vi "Test_Code.vi"() -> ()   [LabVIEW 2015]
uses:
  Serial - Settings.ctl
  Serial - XON-XOFF Characters.ctl
  Serial - ASCII Characters.ctl
  <vilib>/Instr/_visa.llb/Select Event Type.ctl
  <vilib>/Instr/_visa.llb/VISA Configure Serial Port (Instr).vi
  Global 5.vi
  <vilib>/Utility/NIReport.llb/NI_report.lvclass
  <instrlib>/Agilent N6700 Series/Agilent N6700 Series.lvlib
  <vilib>/addons/_office/NI_ReportGenerationToolkit.lvlib
panel:
  in  "report file path":path=path "C:/Users/Tulio/Documents/Testes/Backup excel/backup excel.xlsx"
  out "Hour":i32
  out "Minute":i32
  out "Second":i32
  out "Fractional Second":dbl format="%#.4g"
  in  "Negative Voltage Limit (0.0 volts)":dbl format="%^.3e"
  out "Waveform Graph":dbl[](graph)
  out "Count":i32
  out "read buffer":string
  in  "Read Count":u32=1000
  out "Action":string
  in  "Termination Character":u8=10 format="%.0x"
  in  "End Write on Termination Character?":bool=TRUE
  in  "VISA resource name 2":refnum<visa-resource-name>="COM27"
  in  "XON/XOFF Characters":T1={"XON"=enum."DC1", "XOFF"=enum."DC3"}
  in  "Serial Settings":T3={"baud rate"=9600, "data bits"=8, "parity"=enum."None", "stop bits"=10, "flow control"=0} {"flow control" items=["None"=0, "XON/XOFF"=1, "RTS/CTS"=2, "DTR/DSR"=4]; "stop bits" items=["1.0"=10, "1.5"=15, "2.0"=20]; "data bits" min=5 max=8 step=1; "baud rate" items=["75"=75, "110"=110, "134"=134, "150"=150, "300"=300, "600"=600, "1200"=1200, "1800"=1800, "2400"=2400, "4800"=4800, "7200"=7200, "9600"=9600, "14400"=14400, "19200"=19200, "28800"=28800, "38400"=38400, "56000"=56000, "57600"=57600, "115200"=115200, "128000"=128000, "230400"=230400]}
  in  "End Read on Termination Character?":bool=TRUE
  in  "Start":bool
  in  "Priority (1: Voltage)":i32(ring) items=["Voltage"=1, "Current"=0]
  out "Current Measurement":dbl format="%^.3e"
  in  "Positive Voltage Limit  (5.0 V)":dbl=5.0 format="%^.3e"
  in  "Channel Name (1)":string="4"
  in  "VISA resource name":refnum<visa-resource-name>="USB0::0x0957::0x0F07::MY53002228::INSTR"
  in  "stop":bool
  # "SERIAL"
  # "POWER ANALYZER"
  # "EXCEL"
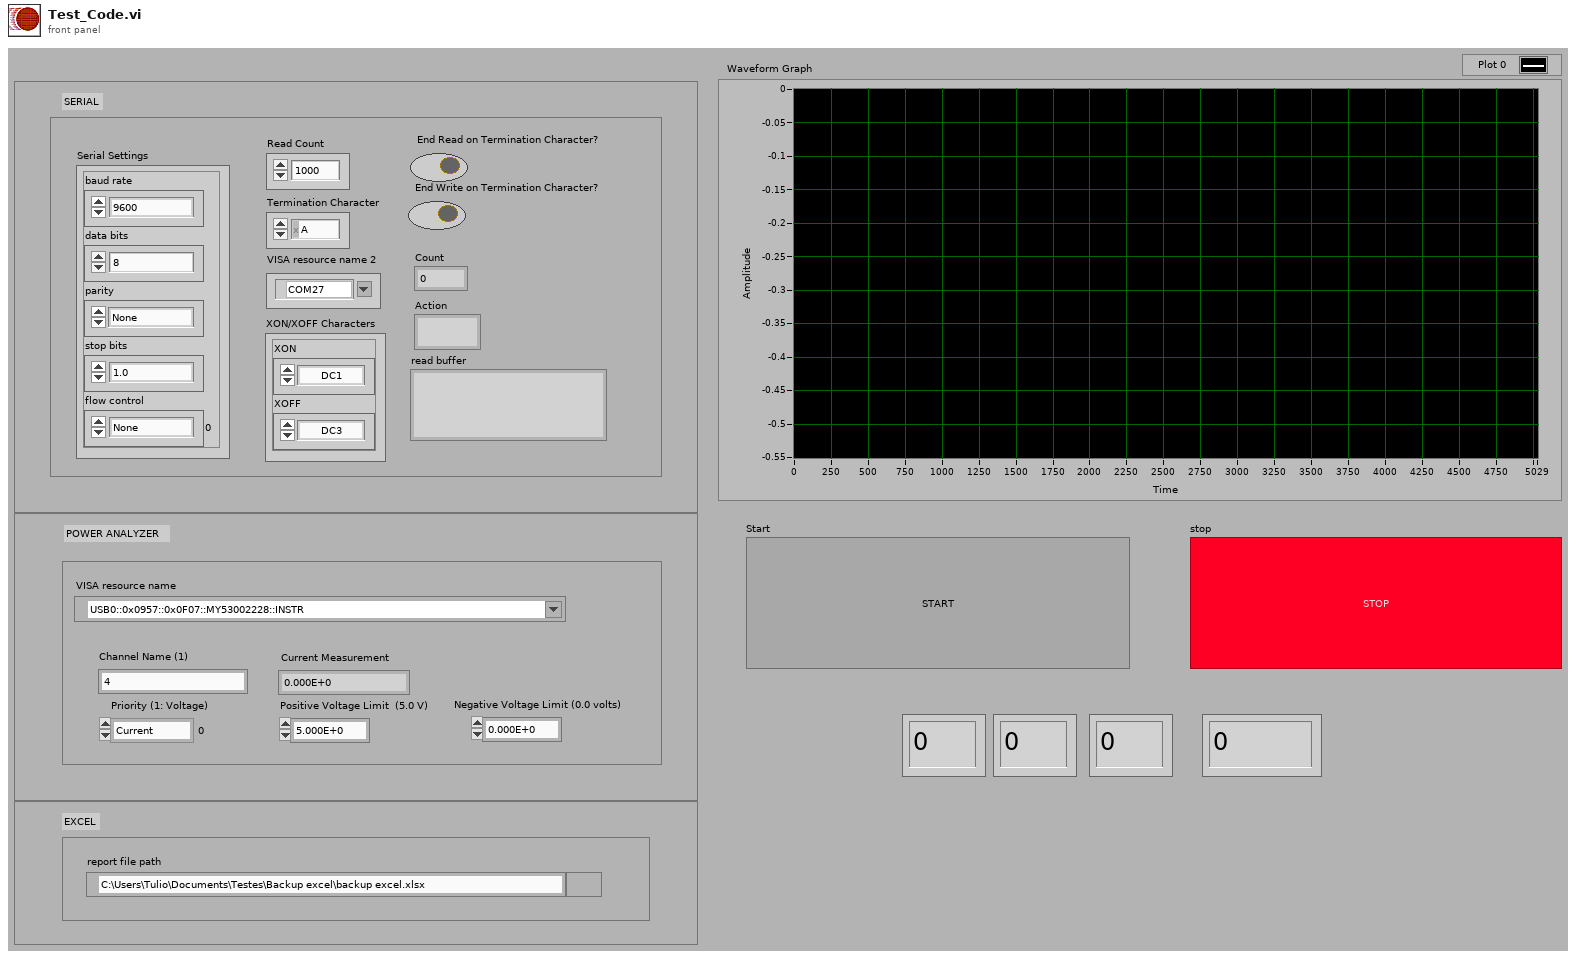
[diagram p1: front panel]
types:
  T1 = typedef "Serial - XON-XOFF Characters.ctl" = cluster{"XON":T2, "XOFF":T2}
  T2 = typedef "Serial - ASCII Characters.ctl" = enum16{"NUL", "SOH", "STX", "ETX", "EOT", "ENQ", "ACK", "BEL", "BS", "HT", "LF", "VT", "FF", "CR", "SO", "SI", "DLE", "DC1", "DC2", "DC3", "DC4", "NAK", "SYN", "ETB", "CAN", "EM", "SUB", "ESC", "FS", "GS", "RS", "US", "SP", "!", "\"", "#", "$", "%", "&", "'", "(", ")", "*", "+", ",", "- (-)", ".", "/", "0", "1", "2", "3", "4", "5", "6", "7", "8", "9", ":", ";", "<", "=", ">", "?", "@", "A", "B", "C", "D", "E", "F", "G", "H", "I", "J", "K", "L", "M", "N", "O", "P", "Q", "R", "S", "T", "U", "V", "W", "X", "Y", "Z", "[", "\\", "]", "^", "_", "`", "a", "b", "c", "d", "e", "f", "g", "h", "i", "j", "k", "l", "m", "n", "o", "p", "q", "r", "s", "t", "u", "v", "w", "x", "y", "z", "{", "|", "}", "~"}
  T3 = typedef "Serial - Settings.ctl" = cluster{"baud rate":u32, "data bits":u16, "parity":enum16{"None", "Odd", "Even", "Mark", "Space"}, "stop bits":u16, "flow control":u16}
  T4 = enum16{"Standard Report", "HTML", "Word", "Excel"}
  T5 = cluster{"Start":bool, "Pause":bool, "Reset":bool}
  T6 = typedef "Select Event Type.ctl" = u32
  T7 = typedef "LVDateTimeRec.ctl" = cluster{"fractional second":dbl, "second":i32, "minute":i32, "hour":i32, "day of month":i32, "month":i32, "year":i32, "day of week":i32, "day of year":i32, "DST":i32}
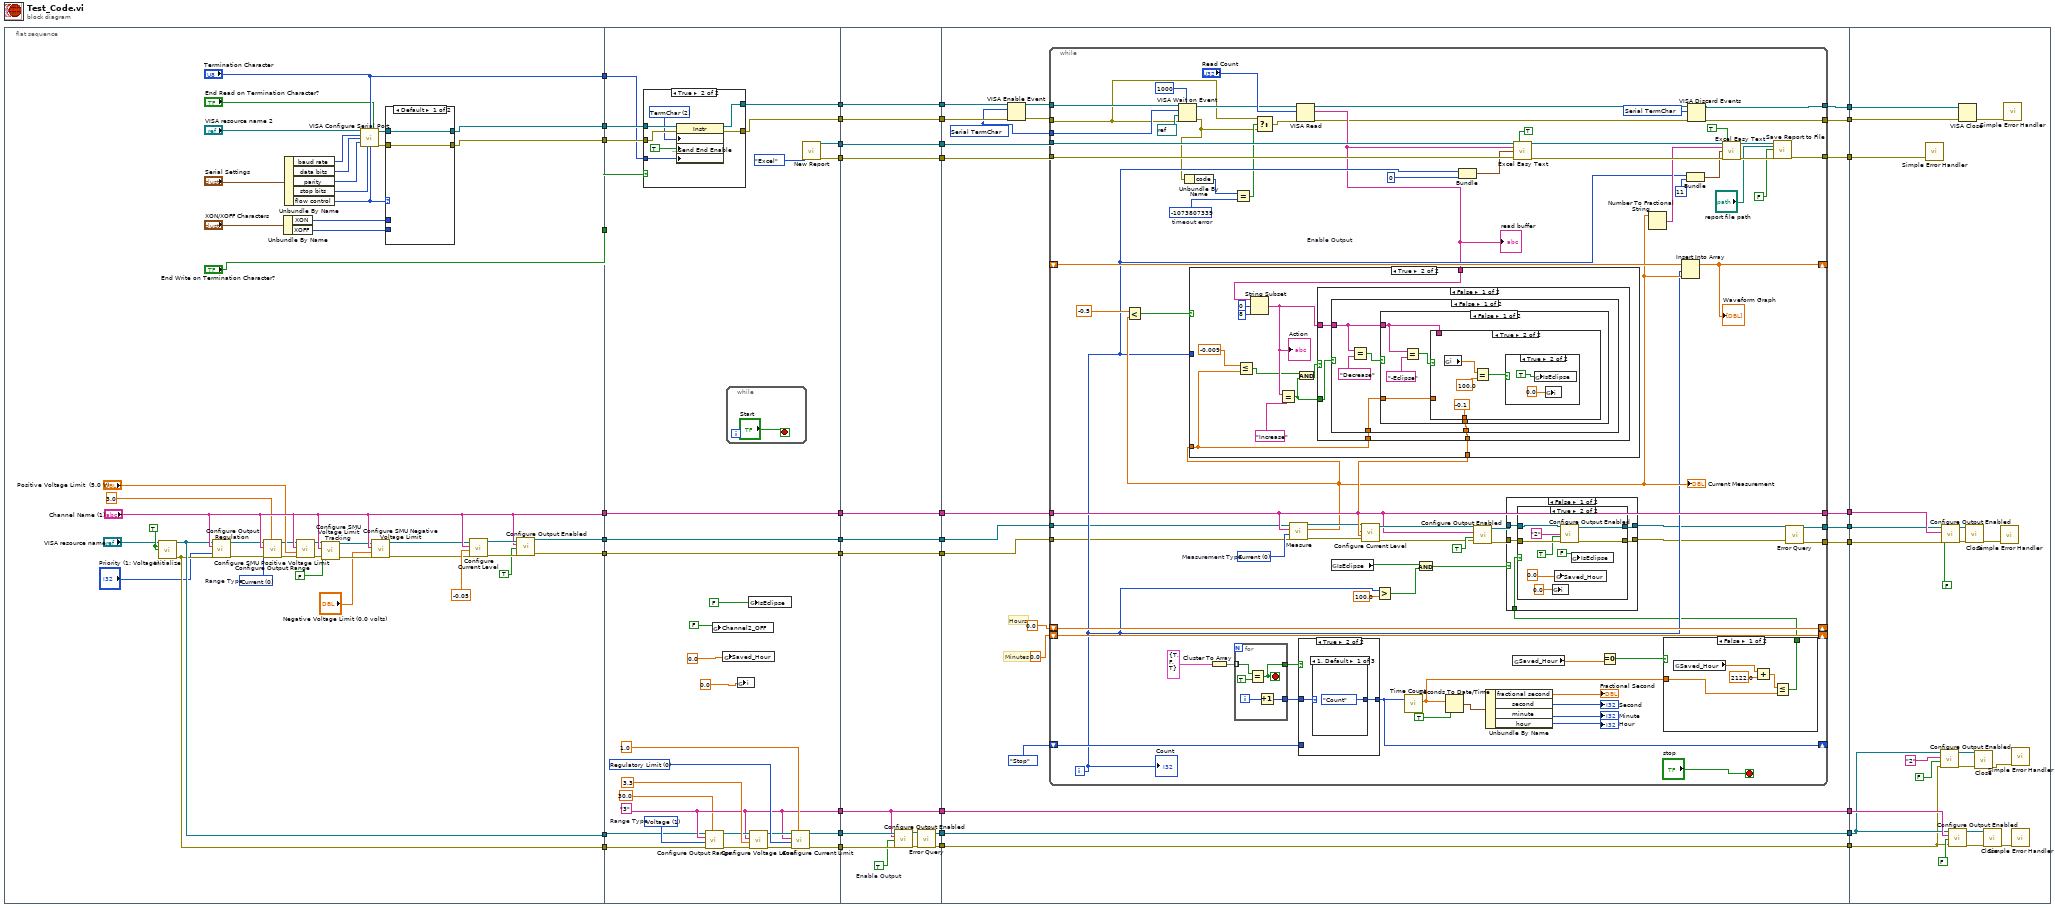
[diagram p0: block diagram]
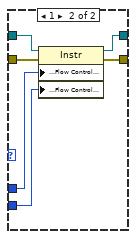
[diagram p2: hidden frame]
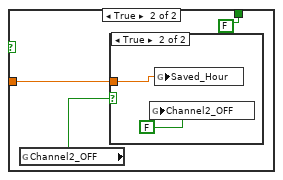
[diagram p4: hidden frame]
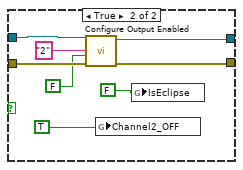
[diagram p7: hidden frame]
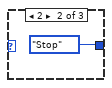
[diagram p9: hidden frame]
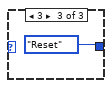
[diagram p10: hidden frame]
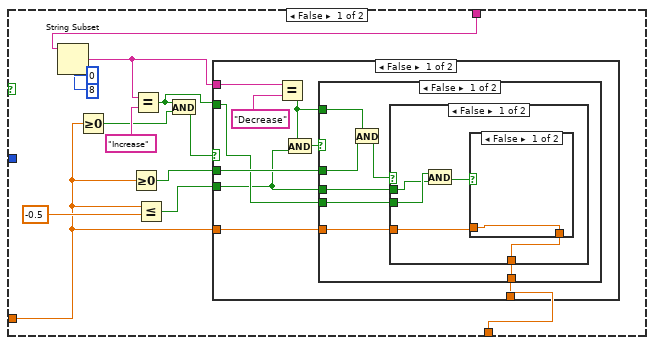
[diagram p11: hidden frame]
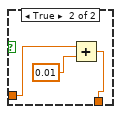
[diagram p12: hidden frame]
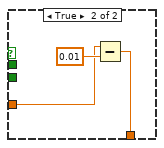
[diagram p13: hidden frame]
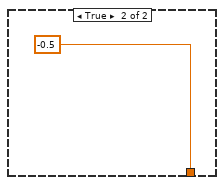
[diagram p14: hidden frame]
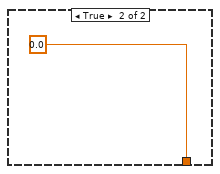
[diagram p15: hidden frame]
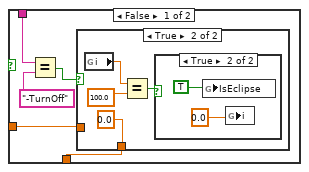
[diagram p16: hidden frame]
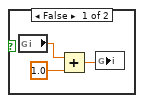
[diagram p18: hidden frame]
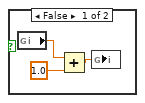
[diagram p19: hidden frame]
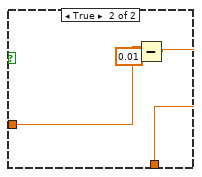
[diagram p20: hidden frame]
diagram:
  n1 = flat-sequence {
    tunnel: ["Channel Name (1)"] -> w38
    tunnel: [w80] -> w37
    tunnel: [w79] -> w36
    tunnel: [w72] -> w35
    tunnel: [w71] -> w34
    tunnel: [w76] -> w25
    tunnel: [w75] -> w24
    tunnel: ["End Write on Termination Character?"] -> w23
    tunnel: ["Termination Character"] -> w22
    tunnel: [w98] -> w20
    tunnel: [w120] -> w18
    tunnel: w38 -> [w120]
    tunnel: [w119] -> w16
    tunnel: w37 -> [w119]
    tunnel: [w118] -> w14
    tunnel: w36 -> [w118]
    tunnel: w35 -> [w99]
    tunnel: w34 -> [w101]
    tunnel: [w109] -> w11
    tunnel: w25 -> [w108]
    tunnel: w24 -> [w107]
    tunnel: w23 -> [w106]
    tunnel: w22 -> [w105]
    tunnel: [w97] -> w9
    tunnel: [w103] -> w7
    tunnel: [w102] -> w5
    tunnel: [w96] -> w2
    tunnel: [w95] -> w1
    tunnel: w20 -> [w145]
    tunnel: [w145] -> w19
    tunnel: w18 -> [w144]
    tunnel: [w144] -> w17
    tunnel: w16 -> [w143]
    tunnel: [w143] -> w15
    tunnel: w14 -> [w142]
    tunnel: [w142] -> w13
    tunnel: [w137] -> w12
    tunnel: w11 -> [w131]
    tunnel: [w131] -> w10
    tunnel: w9 -> [w141]
    tunnel: [w141] -> w8
    tunnel: w7 -> [w140]
    tunnel: [w140] -> w6
    tunnel: w5 -> [w139]
    tunnel: [w139] -> w4
    tunnel: [w138] -> w3
    tunnel: w2 -> [w134]
    tunnel: w1 -> [w133]
    tunnel: w19 -> [w151]
    tunnel: w17 -> [w167]
    tunnel: w15 -> [w166]
    tunnel: w13 -> [w165]
    tunnel: [w164] -> w33
    tunnel: [w163] -> w32
    tunnel: [w162] -> w31
    tunnel: [w161] -> w30
    tunnel: [w160] -> w29
    tunnel: w12 -> [w160]
    tunnel: w10 -> [w159]
    tunnel: [w159] -> w28
    tunnel: [w146] -> w27
    tunnel: [w158] -> w26
    tunnel: w8 -> [w150]
    tunnel: w6 -> [w154]
    tunnel: w4 -> [w153]
    tunnel: [w152] -> w21
    tunnel: w3 -> [w161]
    tunnel: w26 -> [w401]
    tunnel: w27 -> [w402]
    tunnel: w28 -> [w404]
    tunnel: w29 -> [w396]
    tunnel: w30 -> [w397]
    tunnel: w31 -> [w409]
    tunnel: w32 -> [w392]
    tunnel: w33 -> [w391]
    tunnel: w21 -> [w393]
    frame #0 {
      w63 = TRUE ("Reset? (T: Yes)")
      w62 = 0 items=["Voltage"=1, "Current"=0]  # Range Type
      n2 = call <instrlib>:"Initialize.vi"("VISA resource name"="VISA resource name", "ID Query? (T: Yes)"=w63, "Reset? (T: Yes)"=w63) -> ("VISA resource name out"=w72:refnum<visa-resource-name>, "error out"=w71:errorcluster)  [unwired: 11 in]
      n3 = call <instrlib>:"Configure Output Regulation.vi"("VISA resource name"=w72, "Channel Name (1)"="Channel Name (1)", "Output Regulation Priority (1: Voltage)"="Priority (1: Voltage)", "error in (no error)"=w71) -> ("VISA resource name out"=w64:refnum<visa-resource-name>, "error out"=w65:errorcluster)  [unwired: 10 in]
      n4 = call <instrlib>:"Configure Output Range.vi"("Range (0.0)"=3.0, "error in (no error)"=w65, "Range Type (1: Voltage)"=w62, "Channel Name (1)"="Channel Name (1)", "VISA resource name"=w64) -> ("error out"=w67:errorcluster, "VISA resource name out"=w66:refnum<visa-resource-name>)  [unwired: 5 in]
      n5 = Unbundle By Name("XON/XOFF Characters") -> ("XON"=w55:T2, "XOFF"=w56:T2)
      n6 = Unbundle By Name("Serial Settings") -> ("baud rate"=w51:u32, "data bits"=w50:u16, "parity"=w49:enum16{"None", "Odd", "Even", "Mark", "Space"}, "stop bits"=w48:u16, "flow control"=w54:u16)
      n7 = call <instrlib>:"Configure SMU Positive Voltage Limit.vi"("error in (no error)"=w67, "Positive Voltage Limit (0.0 volts)"="Positive Voltage Limit  (5.0 V)", "Channel Name (1)"="Channel Name (1)", "VISA resource name"=w66) -> ("error out"=w69:errorcluster, "VISA resource name out"=w68:refnum<visa-resource-name>)  [unwired: 6 in]
      n8 = call <instrlib>:"Configure SMU Voltage Limit Tracking.vi"("error in (no error)"=w69, "Enable Voltage Limit Tracking (False)"=FALSE, "Channel Name (1)"="Channel Name (1)", "VISA resource name"=w68) -> ("error out"=w42:errorcluster, "VISA resource name out"=w43:refnum<visa-resource-name>)  [unwired: 6 in]
      n9 = call-poly "VISA Configure Serial Port"("VISA resource name"="VISA resource name 2", "termination char\n(0xA = '\\n' = LF)"="Termination Character", "Enable Termination\nChar (T)"="End Read on Termination Character?", "baud rate (9600)"=w51, "data bits (8)"=w50, "parity (0:none)"=w49, "stop bits (10: 1 bit)"=w48, "flow control (0:none)"=w54) -> ("VISA resource name out"=w47:refnum<visa-resource-name>, "error out"=w46:errorcluster)  [unwired: 2 in, 4 out]
      n10 = call <instrlib>:"Configure SMU Negative Voltage Limit.vi"("error in (no error)"=w42, "Negative Voltage Limit (0.0 volts)"="Negative Voltage Limit (0.0 volts)", "Channel Name (1)"="Channel Name (1)", "VISA resource name"=w43) -> ("error out"=w39:errorcluster, "VISA resource name out"=w40:refnum<visa-resource-name>)  [unwired: 6 in]
      n11 = case shown="Default" w54 {
        tunnel: [w83 w90] -> w75
        tunnel: [w84 w89] -> w76
        tunnel: w46 -> [w83 w88]
        tunnel: w47 -> [w84 w87]
        tunnel: w55 -> [_ w86]
        tunnel: w56 -> [_ w85]
        frame Default {
        }
        frame 1 {
          n12 = property class="Instr"(reference=w87, error in=w88, "Serial Settings:Flow Control XON Character"=w86, "Serial Settings:Flow Control XOFF Character"=w85) -> (reference out=w89:refnum<visa-resource-name>, error out=w90:errorcluster)
        }
      }
      n13 = call <instrlib>:"Configure Current Level.vi"("error in (no error)"=w39, "Level  (0.0 A)"=-0.05, "Channel Name (1)"="Channel Name (1)", "VISA resource name"=w40) -> ("error out"=w81:errorcluster, "VISA resource name out"=w82:refnum<visa-resource-name>)  [unwired: 6 in]
      n14 = call <instrlib>:"Configure Output Enabled.vi"("error in (no error)"=w81, "Enable Output (False)"=TRUE, "Channel Name (1)"="Channel Name (1)", "VISA resource name"=w82) -> ("error out"=w79:errorcluster, "VISA resource name out"=w80:refnum<visa-resource-name>)  [unwired: 6 in]
    }
    frame #1 {
      w109 = "3" ("Channel Name (1)")
      w116 = 0 items=["Regulatory Limit", "Trip Limit"] ("Behavior (0: Regulatory Limit)")
      w112 = 1 items=["Voltage"=1, "Current"=0]  # Range Type
      n15 = case shown="True" w106 {
        tunnel: w108 -> [w121 w129]
        tunnel: w107 -> [w122 w128]
        tunnel: [w121 w127] -> w98
        tunnel: [w122 w126] -> w97
        tunnel: w105 -> [_ w124]
        frame False {
        }
        frame True {
          w125 = u16 2 items=["None", "LastBit", "TermChar", "Break"] ("Serial Settings:Serial End Mode for Writes")
          n16 = property class="Instr"(reference=w129, error in=w128, "Serial Settings:End Mode for Writes"=w125, "Message Based Settings:Send End Enable"=TRUE, "Message Based Settings:Termination Character"=w124) -> (reference out=w127:refnum<visa-resource-name>, error out=w126:errorcluster)
        }
      }
      n17 = call <instrlib>:"Configure Output Range.vi"("Range (0.0)"=30.0, "error in (no error)"=w101, "Range Type (1: Voltage)"=w112, "Channel Name (1)"=w109, "VISA resource name"=w99) -> ("error out"=w114:errorcluster, "VISA resource name out"=w113:refnum<visa-resource-name>)  [unwired: 5 in]
      n18 = global write "Global 5.vi" "Channel2_OFF"(FALSE ("Boolean")) -> ()
      n19 = global write "Global 5.vi" "Saved_Hour"(0.0 ("Numeric")) -> ()
      n20 = while {
        stop <- "Start" stop-if-true
      }
      n21 = global write "Global 5.vi" "i"(0.0 ("i")) -> ()
      n22 = global write "Global 5.vi" "IsEclipse"(FALSE ("Boolean")) -> ()
      n23 = call <instrlib>:"Configure Voltage Level.vi"("error in (no error)"=w114, "Level  (0.0 volts)"=3.3, "Channel Name (1)"=w109, "VISA resource name"=w113) -> ("error out"=w110:errorcluster, "VISA resource name out"=w111:refnum<visa-resource-name>)  [unwired: 6 in]
      n24 = call <instrlib>:"Configure Current Limit.vi"("Limit (0.0 amps)"=1.0, "error in (no error)"=w110, "Behavior (0: Regulatory Limit)"=w116, "Channel Name (1)"=w109, "VISA resource name"=w111) -> ("error out"=w95:errorcluster, "VISA resource name out"=w96:refnum<visa-resource-name>)  [unwired: 5 in]
      n25 = call <vilib>:"New Report.vi"("report type"=T4."Excel") -> ("report out"=w103:refnum<class "NI_report.lvclass">, "error out"=w102:errorcluster)  [unwired: 13 in]
    }
    frame #2 {
      w132 = TRUE  # Enable Output
      n26 = call <instrlib>:"Configure Output Enabled.vi"("error in (no error)"=w133, "Enable Output (False)"=w132, "Channel Name (1)"=w131, "VISA resource name"=w134) -> ("error out"=w136:errorcluster, "VISA resource name out"=w135:refnum<visa-resource-name>)  [unwired: 6 in]
      n27 = call <instrlib>:"Error Query.vi"("VISA resource name"=w135, "error in (no error)"=w136) -> ("VISA resource name out"=w138:refnum<visa-resource-name>, "error out"=w137:errorcluster)  [unwired: 10 in, 2 out]
    }
    frame #3 {
      w147 = T6 1073684516 items=["Service Request"=1073684491, "Trigger"=3221168138, "Clear"=1073684493, "VXI Signal"=1073684512, "VXI/VME Interrupt"=3221168161, "VXI/VME Sysfail"=1073684509, "VXI/VME Sysreset"=1073684510, "GPIB CIC"=1073684498, "GPIB Talk"=1073684499, "GPIB Listen"=1073684500, "PXI Interrupt"=1073684514, "Serial Break"=1073684515, "Serial TermChar"=1073684516, "Serial CTS"=1073684521, "Serial DSR"=1073684522, "Serial DCD"=1073684524, "Serial RI"=1073684526, "Serial Character"=1073684533, "USB Interrupt"=1073684535, "All Enabled"=1073709055] ("Event Type")
      # "Minutes"
      # "Hours"
      n28 = VISA Enable Event(8:w150, 10:w147, 11:w151) -> (0:w149:errorcluster, 3:w148:refnum<visa-resource-name>)  [unwired: 1 in]
      n29 = while {
        tunnel: w148 -> [w185]
        tunnel: w167 -> [w237]
        tunnel: w166 -> [w188]
        tunnel: w165 -> [w187]
        tunnel: [w203] -> w164
        tunnel: [w204] -> w163
        tunnel: [w237] -> w162
        tunnel: [w180] -> w158
        tunnel: w149 -> [w174]
        shift-right: [w229] -> _
        shift-left: enum16{"Count", "Stop", "Reset"}."Stop" ("Action") -> [w230]
        shift-right: [w228] -> _
        shift-left: 0.0 -> [w228]
        shift-right: [w227] -> _
        shift-left: 0.0 -> [w227]
        tunnel: w154 -> [w226]
        tunnel: w153 -> [w225]
        tunnel: [w209] -> w152
        shift-right: [w215] -> _
        shift-left: _ -> [w214]
        tunnel: w147 -> [w181]
        tunnel: [w179] -> w146
        i -> [w198]
        stop <- "stop" stop-if-true
        w172 = -1073807339  # timeout error
        w176 = T6 1073684516 items=["Service Request"=1073684491, "Trigger"=3221168138, "Clear"=1073684493, "VXI Signal"=1073684512, "VXI/VME Interrupt"=3221168161, "VXI/VME Sysfail"=1073684509, "VXI/VME Sysreset"=1073684510, "GPIB CIC"=1073684498, "GPIB Talk"=1073684499, "GPIB Listen"=1073684500, "PXI Interrupt"=1073684514, "Serial Break"=1073684515, "Serial TermChar"=1073684516, "Serial CTS"=1073684521, "Serial DSR"=1073684522, "Serial DCD"=1073684524, "Serial RI"=1073684526, "Serial Character"=1073684533, "USB Interrupt"=1073684535, "All Enabled"=1073709055] ("Event Type")
        w241 = 0 items=["Voltage"=1, "Current"=0]  # Measurement Type
        w244 = TRUE  # Enable Output
        n30 = VISA Wait on Event(7:u32 1000 ("timeout (0)"), 8:w174, 9:refnum<visa-resource-name> refnum ("event class (Generic Event)"), 10:w181, 11:w185) -> (0:w170:errorcluster, 3:w184:refnum<visa-resource-name>)  [unwired: 2 out]
        n31 = Unbundle By Name(w170) -> ("code"=w173:i32)
        n32 = Cluster To Array(cluster=T5 {"Start"=TRUE, "Pause"=FALSE, "Reset"=TRUE} ("Buttons")) -> (array=w232:bool[])
        n33 = Equal?(x=w173, y=w172) -> (x = y?=w171:bool)
        n34 = for {
          tunnel: w232 -> [w290] mode=indexing
          tunnel: [w288] -> w233
          tunnel: [w287] -> w234
          i -> [w289]
          stop <- w287 stop-if-true
          n35 = Equal?(x=w290, y=TRUE) -> (x = y?=w287:bool)
          n36 = Increment(x=w289) -> (x+1=w288:i32)
        }
        n37 = Select(t=w174, s=w171, f=w170) -> (s? t:f=w175:errorcluster)
        n38 = call <instrlib>:"Measure.vi"("error in (no error)"=w187, "Measurement Type (1: Voltage)"=w241, "Channel Name (1)"=w237, "VISA resource name"=w188) -> ("error out"=w238:errorcluster, "Measurement"=w213:dbl, "VISA resource name out"=w239:refnum<visa-resource-name>)  [unwired: 5 in]
        "Current Measurement" <- w213
        n39 = Less?(x=-0.5, y=w213) -> (x < y?=w236:bool)
        n40 = VISA Read(VISA resource name=w184, byte count="Read Count", error in (no error)=w175) -> (VISA resource name out=w178:refnum<visa-resource-name>, read buffer=w189:string, error out=w177:errorcluster)  [unwired: 1 out]
        "read buffer" <- w189
        n41 = case shown="True" w236 {
          tunnel: [w304 w345] -> w240
          tunnel: w213 -> [w293 w338]
          tunnel: w189 -> [w297 w343]
          tunnel: w198 -> [_ _]
          frame False {
            n42 = String Subset(string=w297, offset (0)=0, length (rest)=8 ("length (rest)")) -> (substring=w296:string)
            n43 = Greater Or Equal To 0?(x=w293) -> (x >= 0?=w292:bool)
            n44 = Greater Or Equal To 0?(x=w293) -> (x >= 0?=w295:bool)
            n45 = Equal?(x=w296, y="Increase") -> (x = y?=w294:bool)
            n46 = Less Or Equal?(x=w293, y=-0.5) -> (x <= y?=w301:bool)
            n47 = And(x=w294, y=w292) -> (x .and. y?=w303:bool)
            n48 = case shown="False" w303 {
              tunnel: [w310 0.0] -> w304
              tunnel: w301 -> [w305 _]
              tunnel: w296 -> [w312 _]
              tunnel: w295 -> [w308 _]
              tunnel: w293 -> [w307 _]
              tunnel: w294 -> [w306 _]
              frame False {
                n49 = Equal?(x=w312, y="Decrease") -> (x = y?=w309:bool)
                n50 = And(x=w309, y=w305) -> (x .and. y?=w313:bool)
                n51 = case shown="False" w313 {
                  tunnel: [w317 -0.5] -> w310
                  tunnel: w309 -> [w319 _]
                  tunnel: w308 -> [w318 _]
                  tunnel: w307 -> [w316 _]
                  tunnel: w306 -> [w315 _]
                  tunnel: w305 -> [w314 _]
                  frame False {
                    n52 = And(x=w319, y=w318) -> (x .and. y?=w320:bool)
                    n53 = case shown="False" w320 {
                      tunnel: [w322 w332] -> w317
                      tunnel: w316 -> [w321 w330]
                      tunnel: w315 -> [w325 _]
                      tunnel: w314 -> [w324 _]
                      frame False {
                        n54 = And(x=w325, y=w324) -> (x .and. y?=w323:bool)
                        n55 = case shown="False" w323 {
                          tunnel: [w326 w329] -> w322
                          tunnel: w321 -> [w326 w328]
                          frame False {
                          }
                          frame True {
                            n56 = Add(x=w328, y=0.01) -> (x+y=w329:dbl)
                          }
                        }
                      }
                      frame True {
                        n57 = Subtract(x=w330, y=0.01) -> (x-y=w332:dbl)
                      }
                    }
                  }
                  frame True {
                  }
                }
              }
              frame True {
              }
            }
          }
          frame True {
            n58 = Less Or Equal?(x=-0.009, y=w338) -> (x <= y?=w335:bool)
            n59 = String Subset(string=w343, offset (0)=0, length (rest)=8 ("length (rest)")) -> (substring=w340:string)
            "Action" <- w340
            n60 = Equal?(x=w340, y="Increase") -> (x = y?=w337:bool)
            n61 = And(x=w335, y=w337) -> (x .and. y?=w336:bool)
            n62 = case shown="False" w336 {
              tunnel: [w349 0.0 ("Measurement")] -> w345
              tunnel: w337 -> [w348 _]
              tunnel: w338 -> [w347 _]
              tunnel: w340 -> [w346 _]
              frame False {
                n63 = case shown="False" w348 {
                  tunnel: [w354 w388] -> w349
                  tunnel: w346 -> [w350 _]
                  tunnel: w347 -> [w351 w387]
                  frame False {
                    n64 = Equal?(x=w350, y="Decrease") -> (x = y?=w353:bool)
                    n65 = case shown="False" w353 {
                      tunnel: [w357 w385] -> w354
                      tunnel: w351 -> [w356 w384]
                      tunnel: w350 -> [w355 _]
                      frame False {
                        n66 = Equal?(x=w355, y="-Eclipse") -> (x = y?=w359:bool)
                        n67 = case shown="True" w359 {
                          tunnel: [w361 -0.1] -> w357
                          tunnel: w356 -> [w360 _]
                          tunnel: w355 -> [w363 _]
                          frame False {
                            n68 = Equal?(x=w363, y="-TurnOff") -> (x = y?=w364:bool)
                            n69 = case shown="True" w364 {
                              tunnel: [w365 0.0 ("x")] -> w361
                              tunnel: w360 -> [w365 _]
                              frame False {
                              }
                              frame True {
                                n70 = global read "Global 5.vi" "i"() -> (w366:dbl)
                                n71 = Equal?(x=w366, y=100.0) -> (x = y?=w368:bool)
                                n72 = case shown="True" w368 {
                                frame False {
                                n73 = global read "Global 5.vi" "i"() -> (w370:dbl)
                                n74 = Add(x=w370, y=1.0) -> (x+y=w371:dbl)
                                n75 = global write "Global 5.vi" "i"(w371) -> ()
                                }
                                frame True {
                                n76 = global write "Global 5.vi" "IsEclipse"(TRUE ("Boolean")) -> ()
                                n77 = global write "Global 5.vi" "i"(0.0 ("i")) -> ()
                                }
                                }
                              }
                            }
                          }
                          frame True {
                            n78 = global read "Global 5.vi" "i"() -> (w375:dbl)
                            n79 = Equal?(x=w375, y=100.0) -> (x = y?=w377:bool)
                            n80 = case shown="True" w377 {
                              frame False {
                                n81 = global read "Global 5.vi" "i"() -> (w380:dbl)
                                n82 = Add(x=w380, y=1.0) -> (x+y=w379:dbl)
                                n83 = global write "Global 5.vi" "i"(w379) -> ()
                              }
                              frame True {
                                n84 = global write "Global 5.vi" "IsEclipse"(TRUE ("Boolean")) -> ()
                                n85 = global write "Global 5.vi" "i"(0.0 ("i")) -> ()
                              }
                            }
                          }
                        }
                      }
                      frame True {
                        n86 = Subtract(x=w384, y=0.01) -> (x-y=w385:dbl)
                      }
                    }
                  }
                  frame True {
                    n87 = Add(x=w387, y=0.01) -> (x+y=w388:dbl)
                  }
                }
              }
              frame True {
              }
            }
          }
        }
        n88 = case shown="True" w234 {
          tunnel: w233 -> [_ w283]
          tunnel: w230 -> [w281 _]
          tunnel: [w281 w282] -> w229
          frame False {
          }
          frame True {
            n89 = case shown="1, Default" w283 {
              tunnel: [enum16{"Count", "Stop", "Reset"}."Count" ("Action") enum16{"Count", "Stop", "Reset"}."Stop" ("Action") enum16{"Count", "Stop", "Reset"}."Reset" ("Action")] -> w282
              frame 1, Default {
              }
              frame 2 {
              }
              frame 3 {
              }
            }
          }
        }
        n90 = global read "Global 5.vi" "IsEclipse"() -> (w169:bool)
        n91 = call <instrlib>:"Configure Current Level.vi"("error in (no error)"=w238, "Level  (0.0 A)"=w240, "Channel Name (1)"=w237, "VISA resource name"=w239) -> ("error out"=w242:errorcluster, "VISA resource name out"=w243:refnum<visa-resource-name>)  [unwired: 6 in]
        n92 = Greater?(x=w198, y=100.0) -> (0:w200:bool)
        n93 = call "Time Count.vi"("Action"=w229) -> ("Time"=w196:dbl)  [unwired: 10 in]
        n94 = And(x=w169, y=w200) -> (x .and. y?=w197:bool)
        n95 = Seconds To Date/Time(time stamp (now)=w196, to UTC (F)=TRUE) -> (date time rec=w206:T7)
        n96 = Bundle(w198, "offset (0)"=0) -> (w224:cluster{i32, "offset (0)":i32})  [unwired: 1 in]
        n97 = call <instrlib>:"Configure Output Enabled.vi"("error in (no error)"=w242, "Enable Output (False)"=w244, "Channel Name (1)"=w237, "VISA resource name"=w243) -> ("error out"=w201:errorcluster, "VISA resource name out"=w202:refnum<visa-resource-name>)  [unwired: 6 in]
        n98 = Unbundle By Name(w206) -> ("fractional second"=→"Fractional Second":dbl, "second"=→"Second":i32, "minute"=→"Minute":i32, "hour"=→"Hour":i32)
        n99 = global read "Global 5.vi" "Saved_Hour"() -> (w168:dbl)
        n100 = call <vilib>:"Excel Easy Text.vi"("report in"=w226, "border? (F)"=TRUE, "text"=w189, "start (-1, -1)"=w224, "error in (no error)"=w225) -> ("report out"=w221:refnum<class "NI_report.lvclass">, "error out"=w222:errorcluster)  [unwired: 6 in, 3 out]
        n101 = Equal To 0?(x=w168) -> (x = 0?=w195:bool)
        n102 = Number To Fractional String(number=w213) -> (F-format string=w218:string)  [unwired: 3 in]
        n103 = case shown="False" w195 {
          tunnel: w196 -> [w248 w253]
          tunnel: [w250 FALSE] -> w192
          frame False {
            n104 = global read "Global 5.vi" "Saved_Hour"() -> (w247:dbl)
            n105 = Add(x=w247, y=2122.0) -> (x+y=w249:dbl)
            n106 = Less Or Equal?(x=w249, y=w248) -> (x <= y?=w250:bool)
          }
          frame True {
            n107 = global read "Global 5.vi" "Channel2_OFF"() -> (w254:bool)
            n108 = case shown="True" w254 {
              tunnel: w253 -> [_ w255]
              frame False {
              }
              frame True {
                n109 = global write "Global 5.vi" "Channel2_OFF"(FALSE ("Channel2")) -> ()
                n110 = global write "Global 5.vi" "Saved_Hour"(w255) -> ()
              }
            }
          }
        }
        n111 = case shown="False" w197 {
          tunnel: w202 -> [w260 w279]
          tunnel: w201 -> [w261 w278]
          tunnel: [w258 w276] -> w193
          tunnel: [w259 w275] -> w194
          tunnel: w192 -> [w257 _]
          frame False {
            n112 = case shown="True" w257 {
              tunnel: w260 -> [w262 w267]
              tunnel: w261 -> [w263 w271]
              tunnel: [w263 w269] -> w258
              tunnel: [w262 w268] -> w259
              frame False {
              }
              frame True {
                n113 = global write "Global 5.vi" "i"(0.0 ("i")) -> ()
                n114 = global write "Global 5.vi" "Saved_Hour"(0.0 ("Numeric")) -> ()
                n115 = call <instrlib>:"Configure Output Enabled.vi"("error in (no error)"=w271, "Enable Output (False)"=TRUE, "Channel Name (1)"="2", "VISA resource name"=w267) -> ("error out"=w269:errorcluster, "VISA resource name out"=w268:refnum<visa-resource-name>)  [unwired: 6 in]
                n116 = global write "Global 5.vi" "IsEclipse"(FALSE ("Boolean")) -> ()
              }
            }
          }
          frame True {
            n117 = call <instrlib>:"Configure Output Enabled.vi"("error in (no error)"=w278, "Enable Output (False)"=FALSE, "Channel Name (1)"="2", "VISA resource name"=w279) -> ("error out"=w276:errorcluster, "VISA resource name out"=w275:refnum<visa-resource-name>)  [unwired: 6 in]
            n118 = global write "Global 5.vi" "Channel2_OFF"(TRUE ("Channel2")) -> ()
            n119 = global write "Global 5.vi" "IsEclipse"(FALSE ("Boolean")) -> ()
          }
        }
        n120 = Insert Into Array(array=w214, index=w198, new element=w213) -> (w215:dbl[])
        "Waveform Graph" <- w215
        n121 = Bundle(w198, "offset (0)"=11) -> (w219:cluster{i32, "offset (0)":i32})  [unwired: 1 in]
        n122 = VISA Discard Events(8:w177, 10:w176, 11:w178) -> (0:w180:errorcluster, 3:w179:refnum<visa-resource-name>)  [unwired: 1 in]
        n123 = call <vilib>:"Excel Easy Text.vi"("report in"=w221, "border? (F)"=TRUE, "text"=w218, "start (-1, -1)"=w219, "error in (no error)"=w222) -> ("report out"=w211:refnum<class "NI_report.lvclass">, "error out"=w210:errorcluster)  [unwired: 6 in, 3 out]
        n124 = call-dynamic "Save Report to File.vi"("report in"=w211, "report file path"="report file path", "prompt to replace? (F)"=FALSE, "error in (no error)"=w210) -> ("error out"=w209:errorcluster)  [unwired: 10 in, 1 out]
        n125 = call <instrlib>:"Error Query.vi"("VISA resource name"=w194, "error in (no error)"=w193) -> ("VISA resource name out"=w204:refnum<visa-resource-name>, "error out"=w203:errorcluster)  [unwired: 10 in, 2 out]
        "Count" <- w198
      }
    }
    frame #4 {
      n126 = call <vilib>:"Simple Error Handler.vi"("error in (no error)"=w393) -> ()  [unwired: 1 in, 8 out]
      n127 = call <instrlib>:"Configure Output Enabled.vi"("error in (no error)"=w396, "Enable Output (False)"=FALSE, "Channel Name (1)"="2", "VISA resource name"=w397) -> ("error out"=w399:errorcluster, "VISA resource name out"=w400:refnum<visa-resource-name>)  [unwired: 6 in]
      n128 = call <instrlib>:"Configure Output Enabled.vi"("error in (no error)"=w391, "Enable Output (False)"=FALSE, "Channel Name (1)"=w409, "VISA resource name"=w392) -> ("error out"=w411:errorcluster, "VISA resource name out"=w412:refnum<visa-resource-name>)  [unwired: 6 in]
      n129 = call <instrlib>:"Configure Output Enabled.vi"("error in (no error)"=w396, "Enable Output (False)"=FALSE, "Channel Name (1)"=w404, "VISA resource name"=w397) -> ("error out"=w407:errorcluster, "VISA resource name out"=w406:refnum<visa-resource-name>)  [unwired: 6 in]
      n130 = VISA Close(VISA resource name=w402, error in (no error)=w401) -> (error out=w403:errorcluster)
      n131 = call <instrlib>:"Close.vi"("VISA resource name"=w412, "error in (no error)"=w411) -> ("error out"=w413:errorcluster)  [unwired: 13 in]
      n132 = call <instrlib>:"Close.vi"("VISA resource name"=w400, "error in (no error)"=w399) -> ("error out"=w398:errorcluster)  [unwired: 13 in]
      n133 = call <instrlib>:"Close.vi"("VISA resource name"=w406, "error in (no error)"=w407) -> ("error out"=w408:errorcluster)  [unwired: 13 in]
      n134 = call <vilib>:"Simple Error Handler.vi"("error in (no error)"=w413) -> ()  [unwired: 4 in, 5 out]
      n135 = call <vilib>:"Simple Error Handler.vi"("error in (no error)"=w403) -> ()  [unwired: 1 in, 8 out]
      n136 = call <vilib>:"Simple Error Handler.vi"("error in (no error)"=w398) -> ()  [unwired: 4 in, 5 out]
      n137 = call <vilib>:"Simple Error Handler.vi"("error in (no error)"=w408) -> ()  [unwired: 4 in, 5 out]
    }
  }
